vi "test_Create Data Channel_single channel format.vi"(8 "error in (no error)":errorcluster, 11 "TestCase in":refnum<class "Instrument Addon Scripting API Channels Unit Tests.lvclass">) -> (0 "error out":errorcluster, 3 "TestCase out":refnum<class "Instrument Addon Scripting API Channels Unit Tests.lvclass">)   [LabVIEW 2019, in "Instrument Addon Scripting API Channels Unit Tests.lvclass"]
uses:
  Instrument Addon Scripting API Channels Unit Tests.lvclass
  APIs/Scripting API/TypeDefs/Single Channel Format Settings.ctl
  Addon/Addon Shared/Types/Protocol Data Type.ctl
  Addon/Addon Shared/Types/Data Channel Type.ctl
  Instrument Addon Scripting API Channels Unit Tests.lvclass/Instrument Addon Scripting API Channels Unit Tests.ctl
  Addon/Addon Shared/SubVIs/Constants.vi
  <vilib>/NI/NI VeriStand Advanced SysDef API/_SubVIs/SysDef.Search.GUID.vi
  <vilib>/NI/NI VeriStand Advanced SysDef API/_SubVIs/SysDef.Search.GUIDs.vi
  APIs/Scripting API/Channels/Create Data Channel - Single Channel - Format.vi
  <vilib>/NI VeriStand/Custom Device API/Get Item Property (U16).vi
  <vilib>/NI VeriStand/Custom Device API/Get Item Property (String).vi
  <vilib>/addons/_JKI Toolkits/VI Tester/TestCase.llb/TestCase.lvclass
  Instrument Addon Scripting API Test Assets/Instrument Addon Scripting API Test Assets.lvclass
  <vilib>/NI/NI VeriStand Advanced SysDef API/SysDef API/Advanced System Definition.lvlib
  Addon/Addon Shared/Instrument Addon Shared.lvlib
  <vilib>/NI VeriStand/Custom Device API/Custom Device API.lvlib
  APIs/Scripting API/Instrument Addon Scripting API.lvlib
  C:/Program Files (x86)/National Instruments/LabVIEW 2019/vi.lib/addons/_JKI Toolkits/VI Tester/TestCase.llb/TestCase.lvclass
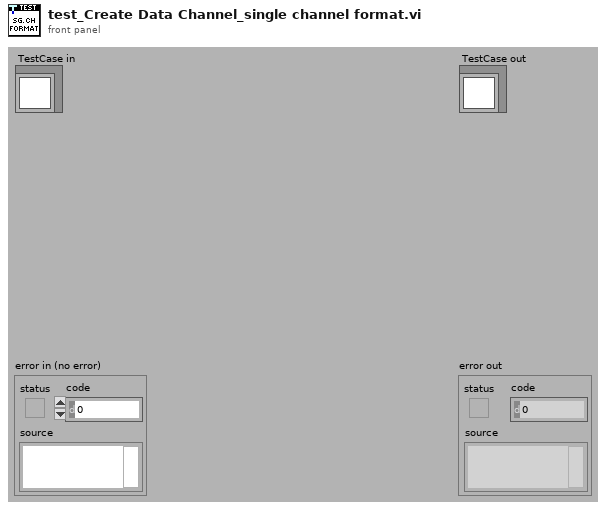
[diagram p1: front panel]
types:
  T1 = typedef "Instrument Addon Scripting API.lvlib/Single Channel Format Settings.ctl" = cluster{"Format String":string, "Default Value":dbl, "Units":string}
  T2 = typedef "Instrument Addon Shared.lvlib/Data Channel Type.ctl" = enum16{"Format", "Comparison", "Type Cast", "Enumerated List"}
  T3 = typedef "Instrument Addon Shared.lvlib/Protocol Data Type.ctl" = enum16{"Single Channel", "Array"}
  T4 = typedef "Custom Device API.lvlib/Custom Device Item Ref.ctl" = u64
  T5 = typedef "Custom Device API.lvlib/Custom Device Channel.ctl" = cluster{"Type":T6, "Units":string, "Default Value":dbl, "Faultable":bool, "Scalable":bool}
  T6 = typedef "Custom Device API.lvlib/Custom Device Channel Type.ctl" = enum16{"Input", "Output"}
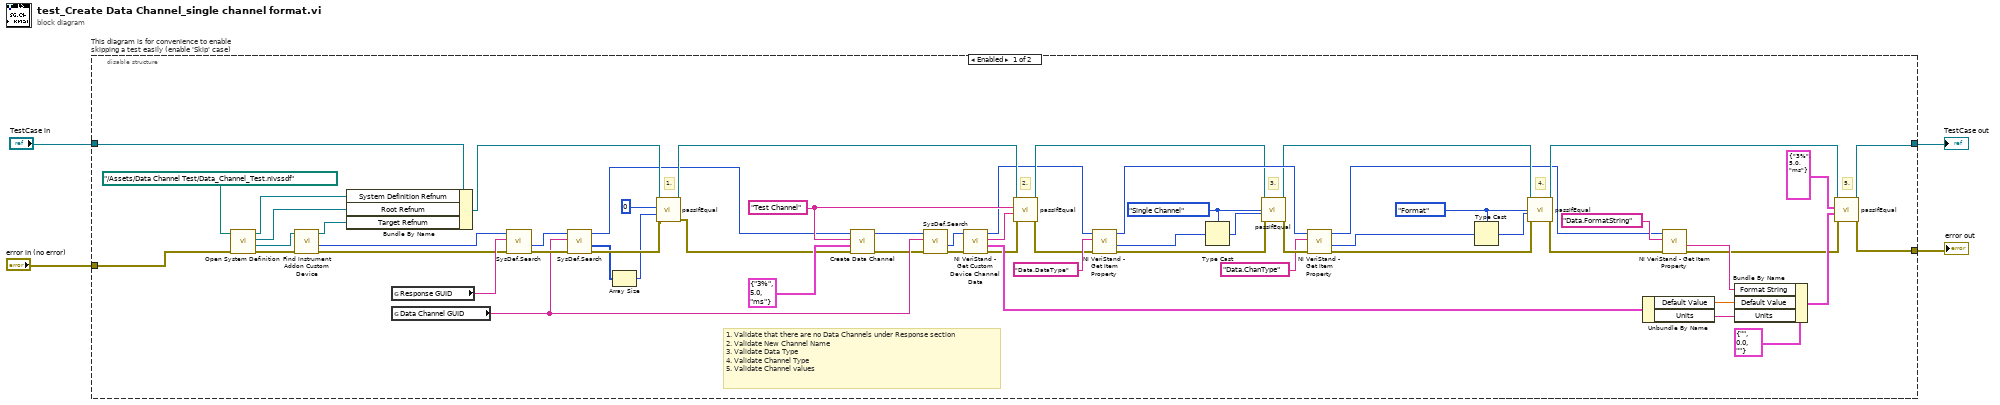
[diagram p0: block diagram]
diagram:
  n1 = disable-structure "This diagram is for convenience to enable skipping a test easily (enable 'Skip' case)" shown="Enabled" {
    disable-tunnel: "TestCase in" -> [w30 w68]
    disable-tunnel: [w64 w66] -> w1
    disable-tunnel: [w63 w67] -> w3
    disable-tunnel: "error in (no error)" -> [w59 w65]
    frame Enabled {
      w16 = Data_Channel_Type."Format" ("Channel Type")
      w21 = Protocol_Data_Type."Single Channel" ("Data Type")
      w41 = "Test Channel" ("Name")
      # "1. Validate that there are no Data Channels under Response section\n2. Validate New Channel Name\n3. Validate Data Type\n4. Validate Channel Type\n5. Validate Channel values"
      # "4."
      # "3."
      # "5."
      # "2."
      # "1."
      n2 = call "Open System Definition.vi"("error in (no error)"=w59, "System Definition File"=path "../Assets/Data Channel Test/Data_Channel_Test.nivssdf") -> ("error out"=w62:errorcluster, "Target Refnum"=w61:refnum<k24>, "Root Refnum"=w33:refnum<k24>, "System Definition Refnum"=w34:refnum<k24>)  [unwired: 6 in]
      n3 = call "Find Instrument Addon Custom Device.vi"("error in"=w62, "target in"=w61) -> ("error out"=w31:errorcluster, "NodeID"=w58:u64, "target out"=w32:refnum<k24>)  [unwired: 7 in]
      n4 = Bundle By Name(cluster=w30, "System Definition Refnum"=w34, "Root Refnum"=w33, "Target Refnum"=w32) -> (w29:refnum<class "Instrument Addon Scripting API Channels Unit Tests.lvclass">)
      n5 = global read "Constants.vi" "Response GUID"() -> (w57:string)
      n6 = global read "Constants.vi" "Data Channel GUID"() -> (w54:string)
      n7 = call-poly <vilib>:"SysDef.Search.vi"("error in (no error)"=w31, "GUID"=w57, "nodeID"=w58) -> ("error out"=w55:errorcluster, "Value out"=w56:u64)  [unwired: 5 in, 2 out]
      n8 = call-poly <vilib>:"SysDef.Search.vi"("error in (no error)"=w55, "GUID"=w54, "nodeID"=w56) -> ("error out"=w45:errorcluster, "Values Out"=w44:u64[], "nodeID out"=w5:u64)  [unwired: 5 in, 1 out]
      n9 = Array Size(array=w44) -> (size(s)=w43:i32)
      n10 = call-dynamic "passIfEqual.vi"("error in (no error)"=w45, "y"=w43, "x"=0 ("size(s)"), "TestCase in"=w29) -> ("error out"=w28:errorcluster, "TestCase out"=w26:refnum<class "Instrument Addon Scripting API Channels Unit Tests.lvclass">)  [unwired: 6 in]
      n11 = call-poly "Create Data Channel.vi"("error in (no error)"=w28, "settings"=T1 {"Format String"="3%", "Default Value"=5.0, "Units"="ms"} ("Settings"), "channel name"=w41, "response refnum in"=w5) -> ("error out"=w39:errorcluster, "response refnum out"=w40:T4)  [unwired: 5 in, 1 out]
      n12 = call-poly <vilib>:"SysDef.Search.vi"("error in (no error)"=w39, "GUID"=w54, "nodeID"=w40) -> ("error out"=w53:errorcluster, "Value out"=w52:u64)  [unwired: 5 in, 2 out]
      n13 = call <vilib>:"NI VeriStand - Get Custom Device Channel Data.vi"("error in (no error)"=w53, "Channel Ref in"=w52) -> ("error out"=w27:errorcluster, "Channel"=w51:T5, "Channel Name"=w47:string, "Channel Ref out"=w7:T4)  [unwired: 4 in, 2 out]
      n14 = call-dynamic "passIfEqual.vi"("error in (no error)"=w27, "y"=w47, "x"=w41, "TestCase in"=w26) -> ("error out"=w13:errorcluster, "TestCase out"=w12:refnum<class "Instrument Addon Scripting API Channels Unit Tests.lvclass">)  [unwired: 6 in]
      n15 = call-poly <vilib>:"NI VeriStand - Get Item Property.vi"("error in (no error)"=w13, "Property Name"="Data.DataType", "Item Ref in"=w7) -> ("error out"=w24:errorcluster, "Value"=w23:u16, "Item Ref out"=w15:T4)  [unwired: 5 in, 1 out]
      n16 = Type Cast(type=w21, x=w23) -> (*(type *) &x=w22:T3)
      n17 = call-dynamic "passIfEqual.vi"("error in (no error)"=w24, "y"=w22, "x"=w21, "TestCase in"=w12) -> ("error out"=w20:errorcluster, "TestCase out"=w11:refnum<class "Instrument Addon Scripting API Channels Unit Tests.lvclass">)  [unwired: 6 in]
      n18 = call-poly <vilib>:"NI VeriStand - Get Item Property.vi"("error in (no error)"=w20, "Property Name"="Data.ChanType", "Item Ref in"=w15) -> ("error out"=w19:errorcluster, "Value"=w18:u16, "Item Ref out"=w6:T4)  [unwired: 5 in, 1 out]
      n19 = Type Cast(type=w16, x=w18) -> (*(type *) &x=w17:T2)
      n20 = call-dynamic "passIfEqual.vi"("error in (no error)"=w19, "y"=w17, "x"=w16, "TestCase in"=w11) -> ("error out"=w10:errorcluster, "TestCase out"=w8:refnum<class "Instrument Addon Scripting API Channels Unit Tests.lvclass">)  [unwired: 6 in]
      n21 = Unbundle By Name(w51) -> ("Default Value"=w50:dbl, "Units"=w49:string)
      n22 = call-poly <vilib>:"NI VeriStand - Get Item Property.vi"("error in (no error)"=w10, "Property Name"="Data.FormatString", "Item Ref in"=w6) -> ("error out"=w9:errorcluster, "Value"=w36:string)  [unwired: 5 in, 2 out]
      n23 = Bundle By Name(cluster=T1 {"Format String"="", "Default Value"=0.0, "Units"=""} ("Settings"), "Format String"=w36, "Default Value"=w50, "Units"=w49) -> (w46:T1)
      n24 = call-dynamic "passIfEqual.vi"("error in (no error)"=w9, "y"=w46, "x"=T1 {"Format String"="3%", "Default Value"=5.0, "Units"="ms"} ("Settings"), "TestCase in"=w8) -> ("error out"=w63:errorcluster, "TestCase out"=w64:refnum<class "Instrument Addon Scripting API Channels Unit Tests.lvclass">)  [unwired: 6 in]
    }
    frame Disabled {
      # "skip test result while test is under development"
      n25 = call <vilib>:"skip.vi"("error in (no error)"=w65, "TestCase in"=w68) -> ("error out"=w67:errorcluster, "TestCase out"=w66:refnum<class "Instrument Addon Scripting API Channels Unit Tests.lvclass">)  [unwired: 8 in]
    }
  }
  "error out" <- w3
  "TestCase out" <- w1
